vi "Q-Lossy.vi"(7 "Queue Type":T2, 8 "error in":errorcluster, 9 "Index":i32=1, 10 "Read Data":T1, 11 "Q Name":string) -> (0 "error out":errorcluster)   [LabVIEW 2016]
uses:
  PSDAQEG_Task Queue Type.ctl
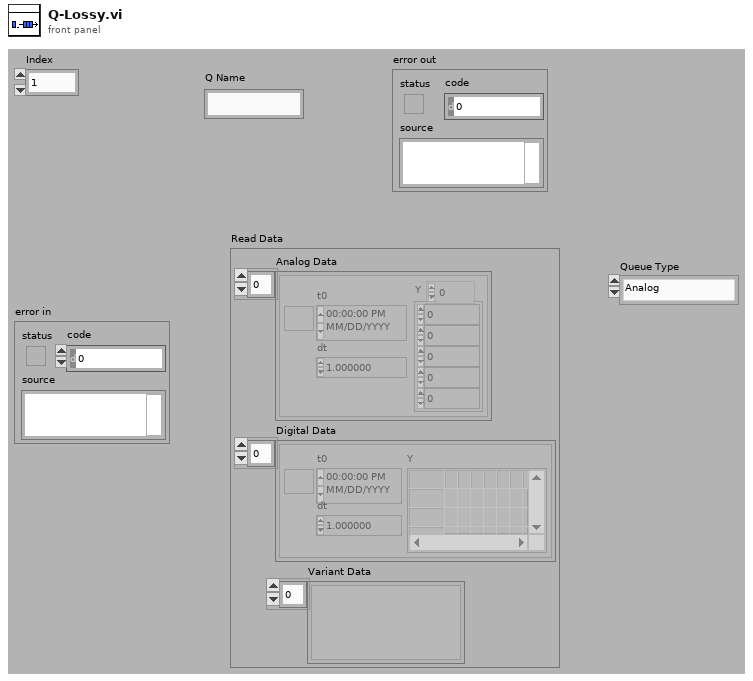
[diagram p1: front panel]
types:
  T1 = cluster{"Analog Data":waveform(dbl)[], "Digital Data":digitalwaveform[], "Variant Data":variant[]}
  T2 = typedef "PSDAQEG_Task Queue Type.ctl" = enum16{"Analog", "Digital", "Variant"}
  T3 = cluster{"Index":i32, "Analog Data":waveform(dbl)[]}
  T4 = cluster{"Index":i32, "Digital Data":digitalwaveform[]}
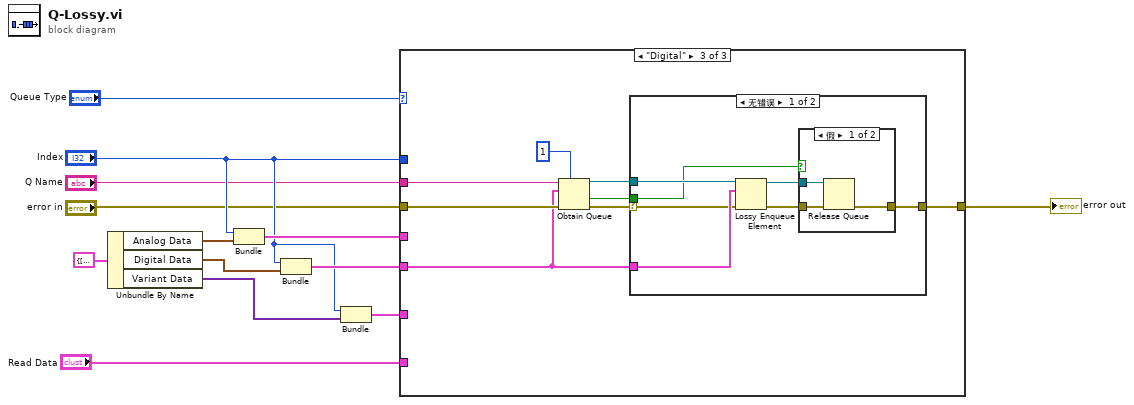
[diagram p0: block diagram]
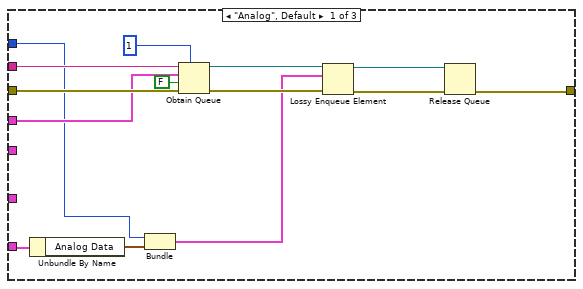
[diagram p2: hidden frame]
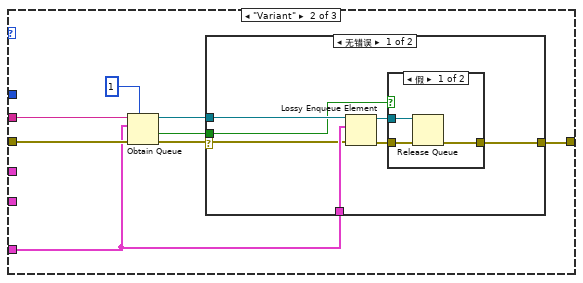
[diagram p3: hidden frame]
diagram:
  n1 = Unbundle By Name(T1 {"Analog Data"=[], "Digital Data"=[], "Variant Data"=[]} ("Read Data")) -> ("Analog Data"=w5:waveform(dbl)[], "Digital Data"=w4:digitalwaveform[], "Variant Data"=w3:variant[])
  n2 = Bundle("Index"="Index", "Analog Data"=w5) -> (w11:T3)  [unwired: 1 in]
  n3 = Bundle("Index"="Index", "Digital Data"=w4) -> (w12:T4)  [unwired: 1 in]
  n4 = Bundle("Index"="Index", "Variant Data"=w3) -> (w9:cluster{"Index":i32, "Variant Data":variant[]})  [unwired: 1 in]
  n5 = case shown="\"Digital\"" "Queue Type" {
    tunnel: "Q Name" -> [w26 w34 w55]
    tunnel: "error in" -> [w27 w35 w54]
    tunnel: "Index" -> [w18 _ _]
    tunnel: w12 -> [_ _ w50]
    tunnel: [w24 w33 w53] -> w8
    tunnel: w11 -> [w23 _ _]
    tunnel: w9 -> [_ w30 _]
    tunnel: "Read Data" -> [w20 _ _]
    frame "Analog", Default {
      n6 = Unbundle By Name(w20) -> ("Analog Data"=w19:waveform(dbl)[])
      n7 = Bundle("Index"=w18, "Analog Data"=w19) -> (w17:T3)  [unwired: 1 in]
      n8 = Obtain Queue(max queue size (-1, unlimited)=1, name (unnamed)=w26, element data type=w23, create if not found? (T)=FALSE, error in (no error)=w27) -> (queue out=w25:refnum<queue>, error out=w21:errorcluster)  [unwired: 1 out]
      n9 = Lossy Enqueue Element(queue=w25, element=w17, error in (no error)=w21) -> (queue out=w15:refnum<queue>, error out=w16:errorcluster)  [unwired: 2 out]
      n10 = Release Queue(queue=w15, error in (no error)=w16) -> (error out=w24:errorcluster)  [unwired: 1 in, 2 out]
    }
    frame "Variant" {
      n11 = Obtain Queue(max queue size (-1, unlimited)=1, name (unnamed)=w34, element data type=w30, error in (no error)=w35) -> (queue out=w32:refnum<queue>, created new?=w31:bool, error out=w28:errorcluster)  [unwired: 1 in]
      n12 = case shown="无错误" w28 {
        selector: w28 -> [w36 w47]
        tunnel: [w40 w47] -> w33
        tunnel: w32 -> [w39 _]
        tunnel: w31 -> [w38 _]
        tunnel: w30 -> [w37 _]
        frame No Error {
          n13 = Lossy Enqueue Element(queue=w39, element=w37, error in (no error)=w36) -> (queue out=w41:refnum<queue>, error out=w42:errorcluster)  [unwired: 2 out]
          n14 = case shown="假" w38 {
            tunnel: w41 -> [w45 _]
            tunnel: w42 -> [w44 w46]
            tunnel: [w43 w46] -> w40
            frame False {
              n15 = Release Queue(queue=w45, error in (no error)=w44) -> (error out=w43:errorcluster)  [unwired: 1 in, 2 out]
            }
            frame True {
            }
          }
        }
        frame Error {
        }
      }
    }
    frame "Digital" {
      n16 = Obtain Queue(max queue size (-1, unlimited)=1, name (unnamed)=w55, element data type=w50, error in (no error)=w54) -> (queue out=w52:refnum<queue>, created new?=w51:bool, error out=w48:errorcluster)  [unwired: 1 in]
      n17 = case shown="无错误" w48 {
        selector: w48 -> [w56 w67]
        tunnel: [w60 w67] -> w53
        tunnel: w52 -> [w59 _]
        tunnel: w51 -> [w58 _]
        tunnel: w50 -> [w57 _]
        frame No Error {
          n18 = Lossy Enqueue Element(queue=w59, element=w57, error in (no error)=w56) -> (queue out=w61:refnum<queue>, error out=w62:errorcluster)  [unwired: 2 out]
          n19 = case shown="假" w58 {
            tunnel: w61 -> [w65 _]
            tunnel: w62 -> [w64 w66]
            tunnel: [w63 w66] -> w60
            frame False {
              n20 = Release Queue(queue=w65, error in (no error)=w64) -> (error out=w63:errorcluster)  [unwired: 1 in, 2 out]
            }
            frame True {
            }
          }
        }
        frame Error {
        }
      }
    }
  }
  "error out" <- w8
